vi "Write Ext.vi"   [LabVIEW 2017, in "LabPack.lvlib" / "Writer.lvclass"]
uses:
  Writer.lvclass
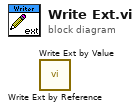
[diagram p0: block diagram]
diagram:
  n1 = call "Write Ext by Reference.vi"() -> ()  [unwired: 10 in, 2 out]
  n2 = call "Write Ext by Value.vi"() -> ()  [unwired: 10 in, 2 out]
